vi "Untitled 1.vi"() -> ()   [LabVIEW 2014]
uses:
  USBAnalyzerEllisysDll/Debug/USBAnalyzerEllisysDll.dll
panel:
  out "tab 2":string
  out "unsigned byte array":u8[](array[numeric])
  in  "tab":string
  out "size 2":i32
  out "return type":i32
  in  "size":i32
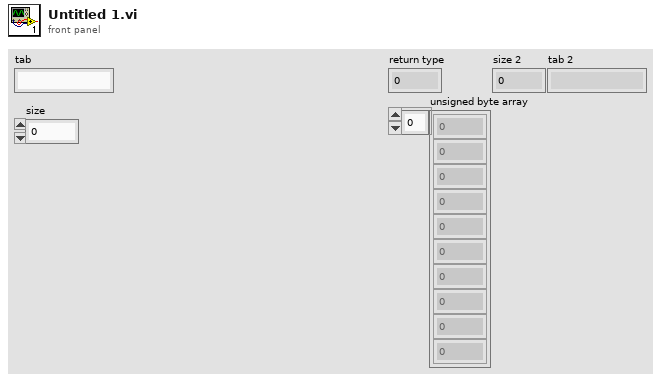
[diagram p1: front panel]
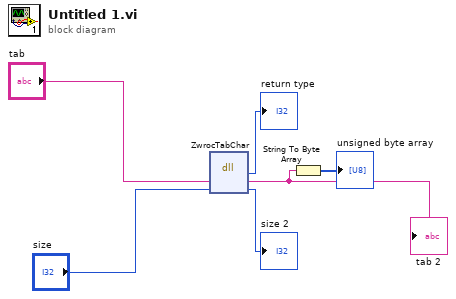
[diagram p0: block diagram]
diagram:
  n1 = dll-call lib="PTH2labs CUsersMichał\tDocumentsEllisysAnalyzerUSBAnalyzerEllisysDllDebugUSBAnalyzerEllisysDll.dll" fn="ZwrocTabChar"("tab"="tab", "size"="size") -> ("return type"=→"return type":i32, "tab"=w2:string, "size"=→"size 2":i32)  [unwired: 3 in, 2 out]
  "tab 2" <- w2
  n2 = String To Byte Array(string=w2) -> (unsigned byte array=→"unsigned byte array":u8[])
